vi "MenuSelection(User).vi"(6 "User events":T8, 7 "Clipboard":refnum<vi>, 8 "error in":errorcluster {"code" min=0 max=0}, 10 "ItemTag":string, 11 "Data in":T1={"Class"={"Ants"=refnum, "Layer"=refnum, "Templates"=refnum, "Icon"=refnum, "Glyph"=refnum, "Settings"=refnum, "Tools"=refnum, "History"=refnum}, "Ref"={"Add Layer"=refnum, "Remove Layer"=refnum, "Line Text"=[], "Body Text Spec"=refnum, "DNL_Font"=refnum, "glyph path str"=refnum, "templates path str"=refnum, "Arrow Up"=refnum, "Arrow Down"=refnum, "IE VI Ref"=refnum, "Glyphs tree"=refnum, "Templates tree"=refnum, "Layer Icon Text"=refnum, "Layer Template"=refnum, "Body Text"=refnum, "Search Templates"=refnum, "TextMarker"=refnum, "Tab Control"=refnum, "Search Glyphs"=refnum, "Line Color"=refnum, "DNL_Glyphs []"=refnum, "Fill Color"=refnum, "Tools"=refnum, "Icon"=refnum, "Preview"=refnum, "Ants"=refnum, "Terminals"=refnum, "menu reference"=refnum, "LayerNames"=[], "GlyphLoadAnimation"=refnum, "TemplateLoadAnimation"=refnum, "refreshGlyphs"=refnum, "refreshTemplates"=refnum}, "Support"={"AntsRect"={"left"=0, "top"=0, "right"=0, "bottom"=0}, "Mouse Move Coords"={"Horizontal"=0, "Vertical"=0}, "Mouse Down Coords"={"Horizontal"=0, "Vertical"=0}, "Temp Coord"={"Horizontal"=0, "Vertical"=0}, "Action"=enum."Default", "Edge Color"=4914962, "Fill Color"=16860, "Mouse Down?"=FALSE, "Draft Mode?"=FALSE, "Temp Icon"=bytes[3102], "CTRL Pressed"=FALSE, "Move Selection?"=FALSE, "AntsRect Orig"={"left"=0, "top"=0, "right"=0, "bottom"=0}, "Text"="", "TM Set?"=FALSE, "Mouse inside icon?"=FALSE, "Tool (old value)"=0, "Pencil Move Color"=0, "Swap Colors?"=FALSE, "Shift pressed?"=FALSE}}) -> (0 "error out":errorcluster {"code" min=0 max=0}, 3 "Data out":T1={"Class"={"Ants"=refnum, "Layer"=refnum, "Templates"=refnum, "Icon"=refnum, "Glyph"=refnum, "Settings"=refnum, "Tools"=refnum, "History"=refnum}, "Ref"={"Add Layer"=refnum, "Remove Layer"=refnum, "Line Text"=[], "Body Text Spec"=refnum, "DNL_Font"=refnum, "glyph path str"=refnum, "templates path str"=refnum, "Arrow Up"=refnum, "Arrow Down"=refnum, "IE VI Ref"=refnum, "Glyphs tree"=refnum, "Templates tree"=refnum, "Layer Icon Text"=refnum, "Layer Template"=refnum, "Body Text"=refnum, "Search Templates"=refnum, "TextMarker"=refnum, "Tab Control"=refnum, "Search Glyphs"=refnum, "Line Color"=refnum, "DNL_Glyphs []"=refnum, "Fill Color"=refnum, "Tools"=refnum, "Icon"=refnum, "Preview"=refnum, "Ants"=refnum, "Terminals"=refnum, "menu reference"=refnum, "LayerNames"=[], "GlyphLoadAnimation"=refnum, "TemplateLoadAnimation"=refnum, "refreshGlyphs"=refnum, "refreshTemplates"=refnum}, "Support"={"AntsRect"={"left"=0, "top"=0, "right"=0, "bottom"=0}, "Mouse Move Coords"={"Horizontal"=0, "Vertical"=0}, "Mouse Down Coords"={"Horizontal"=0, "Vertical"=0}, "Temp Coord"={"Horizontal"=0, "Vertical"=0}, "Action"=enum."Default", "Edge Color"=4914962, "Fill Color"=16860, "Mouse Down?"=FALSE, "Draft Mode?"=FALSE, "Temp Icon"=bytes[3102], "CTRL Pressed"=FALSE, "Move Selection?"=FALSE, "AntsRect Orig"={"left"=0, "top"=0, "right"=0, "bottom"=0}, "Text"="", "TM Set?"=FALSE, "Mouse inside icon?"=FALSE, "Tool (old value)"=0, "Pencil Move Color"=0, "Swap Colors?"=FALSE, "Shift pressed?"=FALSE}})   [LabVIEW 2020]
uses:
  Class/Ants/Ants.lvclass
  Class/FakedArray/FakedArray.lvclass
  vi.lib/LabVIEW Icon API/lv_icon/Classes/Icon/Icon.lvclass
  Class/Icon Library/Glyph.lvclass
  Class/Settings/Settings.lvclass
  Class/Tools/Tools Paint.lvclass
  History/History/History.lvclass
  vi.lib/LabVIEW Icon API/lv_icon/Classes/Icon Framework/Icon Framework.lvclass
  vi.lib/LabVIEW Icon API/lv_icon/Classes/Layer/Layer.lvclass
  vi.lib/LabVIEW Icon API/lv_icon/Controls/Layer.ctl
  Controls/Tools.ctl
  lv_icon.lvlib
  vi.lib/LabVIEW Icon API/LabVIEW Icon API.lvlib
  vi.lib/LabVIEW Icon API/lv_icon/Controls/Pathes.ctl
  History/History.lvlib
  vi.lib/LabVIEW Icon API/lv_icon/Controls/Graphic.ctl
  <vilib>/Utility/miscctls.llb/LVSelectionTypeDef.ctl
  <vilib>/Utility/miscctls.llb/LVPoint32TypeDef.ctl
  Controls/SupportClass_Action.ctl
  vi.lib/LabVIEW Icon API/lv_icon/Controls/IEColor.ctl
  Controls/Support Cluster.ctl
  Controls/References Cluster.ctl
  Controls/IE Classes.ctl
  Controls/Global Data.ctl
panel:
  in  "Layer name":string="Clipboard"
  in  "glyph":string="Glyph name"
  in  "template":string="Template name"
  in  "Prompt":string="Save Glyph"
  in  "prompt":string="Save Icon Template"
  in  "LayerName":string="Merged Layers"
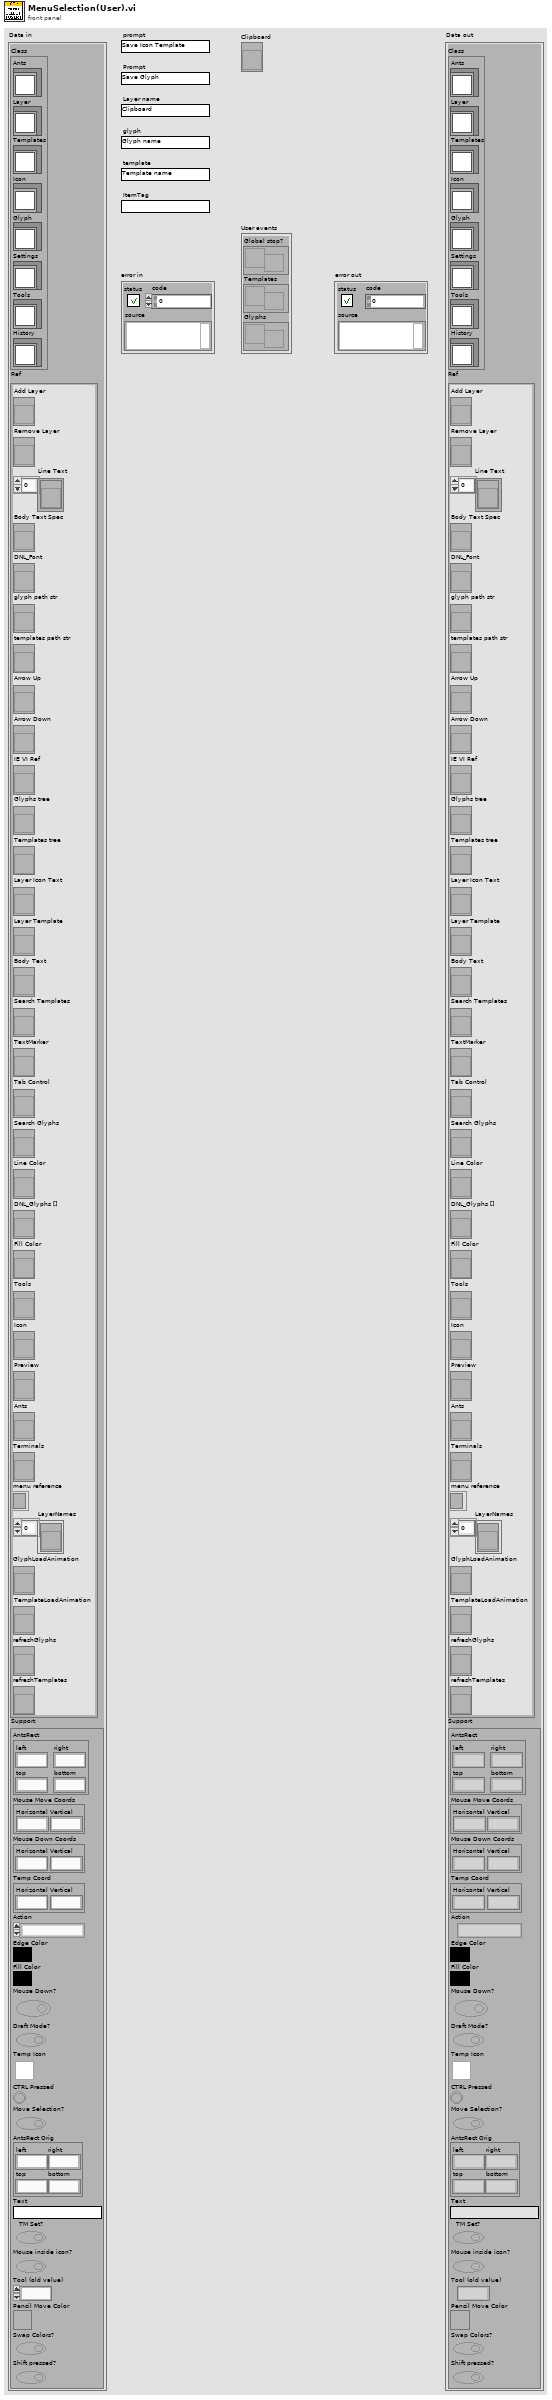
[diagram p1: front panel]
types:
  T1 = typedef "lv_icon.lvlib/Global Data.ctl" = cluster{"Class":T2, "Ref":T3, "Support":T4}
  T2 = typedef "lv_icon.lvlib/IE Classes.ctl" = cluster{"Ants":refnum<class "Ants.lvclass">, "Layer":refnum<class "FakedArray.lvclass">, "Templates":refnum<class "FakedArray.lvclass">, "Icon":refnum<class "Icon.lvclass">, "Glyph":refnum<class "Glyph.lvclass">, "Settings":refnum<class "Settings.lvclass">, "Tools":refnum<class "Tools Paint.lvclass">, "History":refnum<class "History.lvclass">}
  T3 = typedef "lv_icon.lvlib/References Cluster.ctl" = cluster{"Add Layer":refnum<vi>, "Remove Layer":refnum<vi>, "Line Text":refnum<vi>[], "Body Text Spec":refnum<vi>, "DNL_Font":refnum<vi>, "glyph path str":refnum<vi>, "templates path str":refnum<vi>, "Arrow Up":refnum<vi>, "Arrow Down":refnum<vi>, "IE VI Ref":refnum<vi>, "Glyphs tree":refnum<vi>, "Templates tree":refnum<vi>, "Layer Icon Text":refnum<vi>, "Layer Template":refnum<vi>, "Body Text":refnum<vi>, "Search Templates":refnum<vi>, "TextMarker":refnum<vi>, "Tab Control":refnum<vi>, "Search Glyphs":refnum<vi>, "Line Color":refnum<vi>, "DNL_Glyphs []":refnum<vi>, "Fill Color":refnum<vi>, "Tools":refnum<vi>, "Icon":refnum<vi>, "Preview":refnum<vi>, "Ants":refnum<vi>, "Terminals":refnum<vi>, "menu reference":refnum<k9>, "LayerNames":refnum<vi>[], "GlyphLoadAnimation":refnum<vi>, "TemplateLoadAnimation":refnum<vi>, "refreshGlyphs":refnum<vi>, "refreshTemplates":refnum<vi>}
  T4 = typedef "lv_icon.lvlib/Support Cluster.ctl" = cluster{"AntsRect":cluster{"left":i16, "top":i16, "right":i16, "bottom":i16}, "Mouse Move Coords":T5, "Mouse Down Coords":T5, "Temp Coord":T5, "Action":T6, "Edge Color":T7, "Fill Color":T7, "Mouse Down?":bool, "Draft Mode?":bool, "Temp Icon":picture, "CTRL Pressed":bool, "Move Selection?":bool, "AntsRect Orig":cluster{"left":i16, "top":i16, "right":i16, "bottom":i16}, "Text":string, "TM Set?":bool, "Mouse inside icon?":bool, "Tool (old value)":u32, "Pencil Move Color":u32, "Swap Colors?":bool, "Shift pressed?":bool}
  T5 = typedef "LVPoint32TypeDef.ctl" = cluster{"Horizontal":i32, "Vertical":i32}
  T6 = typedef "SupportClass_Action.ctl" = enum16{"Default", "Move Selection", "Glyph Library", "Tool"}
  T7 = typedef "IEColor.ctl" = u32
  T8 = cluster{"Global stop?":refnum<user-event>, "Templates":refnum<user-event>, "Glyphs":refnum<user-event>}
  T9 = typedef "Pathes.ctl" = enum16{"Root Path", "Icon Templates", "Icon Templates VI", "Icon Templates Lib", "Glyphs"}
  T10 = typedef "Graphic.ctl" = cluster{"Rectangle":cluster{"left":i16, "top":i16, "right":i16, "bottom":i16}, "Path":path, "Image":picture, "Filter":string, "FileName":string}
  T11 = typedef "Layer.ctl" = cluster{"LayerIcon":picture, "LayerName":string, "Opacity":u8, "Visibility?":bool}
  T12 = enum32{"Pencil", "Line", "Dropper", "Fill", "Rectangle", "Filled Rectangle", "Ellipse", "Filled Ellipse", "Eraser", "Text", "Select", "Move"}
  T13 = typedef "LVSelectionTypeDef.ctl" = cluster{"Selection Start":u32, "Selection End":u32}
  T14 = typedef "Tools.ctl" = enum32{"Pencil", "Line", "Dropper", "Fill", "Rectangle", "Filled Rectangle", "Ellipse", "Filled Ellipse", "Eraser", "Text", "Select", "Move"}
  T15 = typedef "imagedata.ctl" = cluster{"image type":i32, "image depth":i32, "image":u8[], "mask":u8[], "colors":u32[], "Rectangle":cluster{"left":i16, "top":i16, "right":i16, "bottom":i16}}
  T16 = typedef "Font.ctl" = string
  T17 = typedef "Alignment.ctl" = u16
  T18 = typedef "Font Size.ctl" = u8
  T19 = cluster{"Line 1 text":string, "Line 2 text":string, "Line 3 text":string, "Line 4 text":string, "Line 1 color":u32, "Line 2 color":u32, "Line 3 color":u32, "Line 4 color":u32, "Body Text Spec":cluster{"DNL_Font":T16, "Alignment":T17, "Size":T18}, "Center text vertically":bool, "Capitalize Text":bool}
  T20 = cluster{"left":i16, "top":i16, "right":i16, "bottom":i16}
  T21 = cluster{"Horizontal":i32, "Vertical":i32, "Vertical 2":i32, "Vertical 3":i32}
  T22 = typedef "lv_icon.lvlib/History.lvlib/State.ctl" = cluster{"Template":string, "Layers":string, "Body Text":string, "Icon Text Layer":string, "Template Layer":string, "Templates Search":string, "Glyphs Search":string}
  T23 = cluster{"Left":i32, "Top":i32, "Right":i32, "Bottom":i32}
  T24 = typedef "Icon Editor Invoker Type.ctl" = enum32{"Unknown Icon Source", "VI Icon", "Library Icon (any library type)", "Palette icon", "Icon from App Method"}
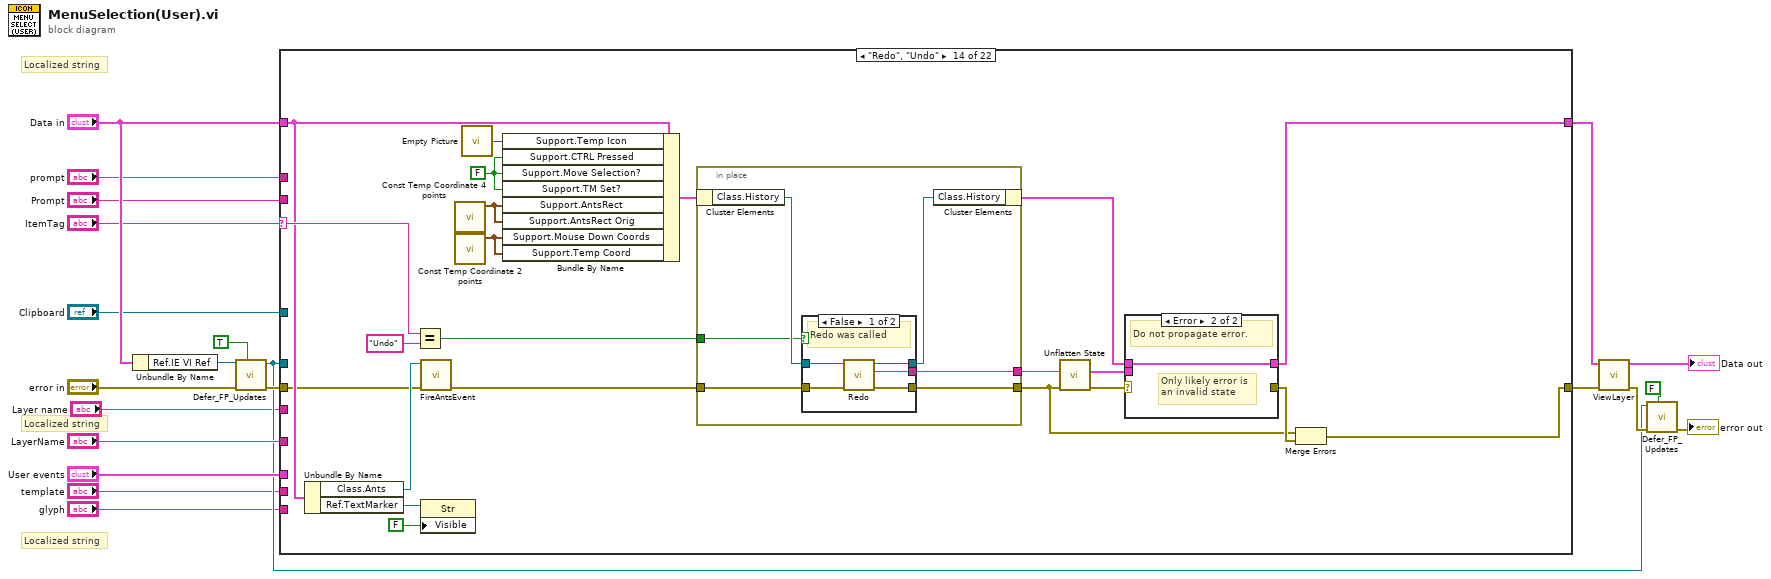
[diagram p0: block diagram]
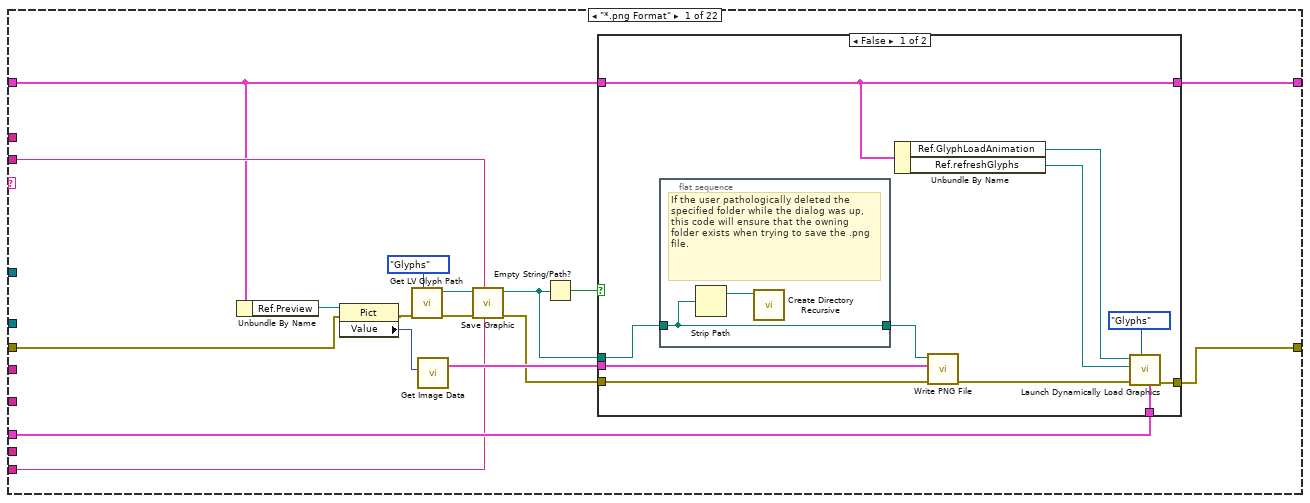
[diagram p2: hidden frame]
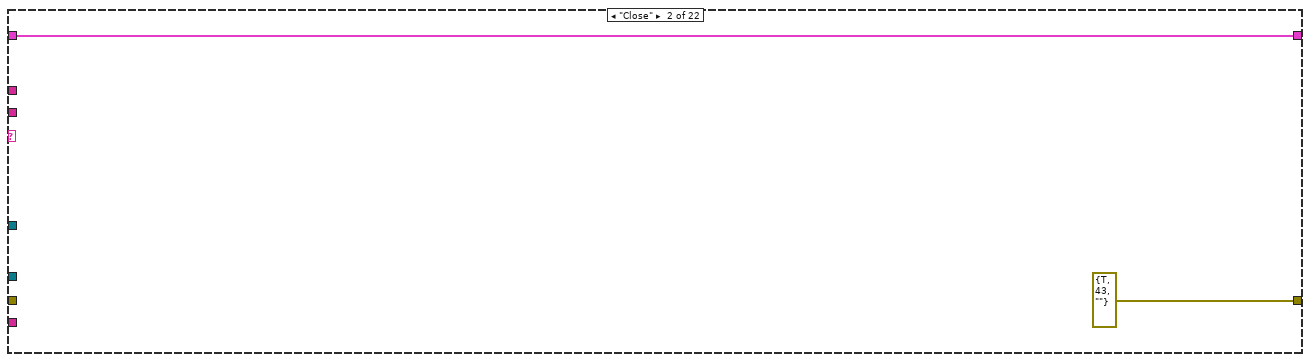
[diagram p4: hidden frame]
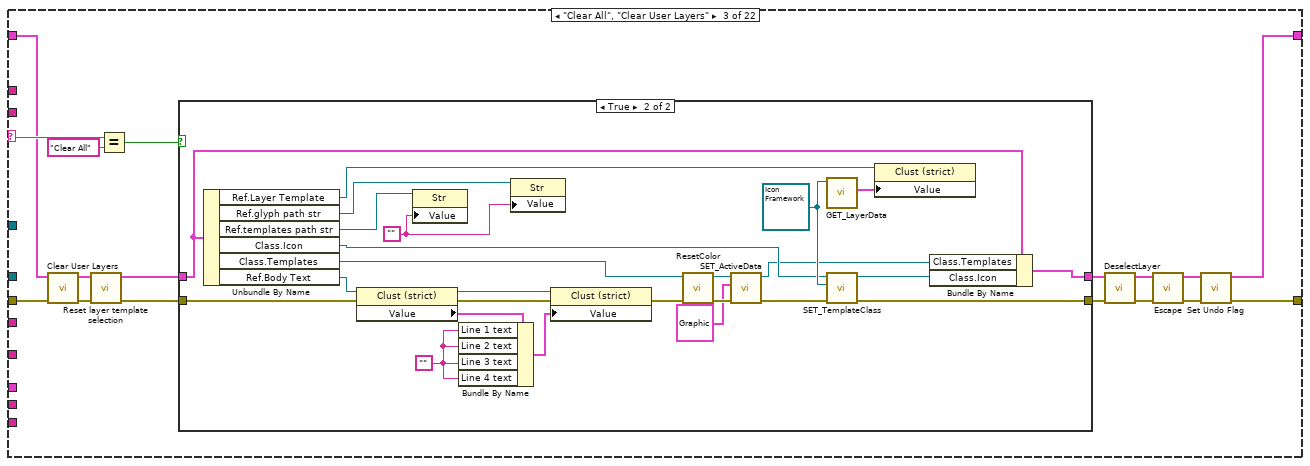
[diagram p5: hidden frame]
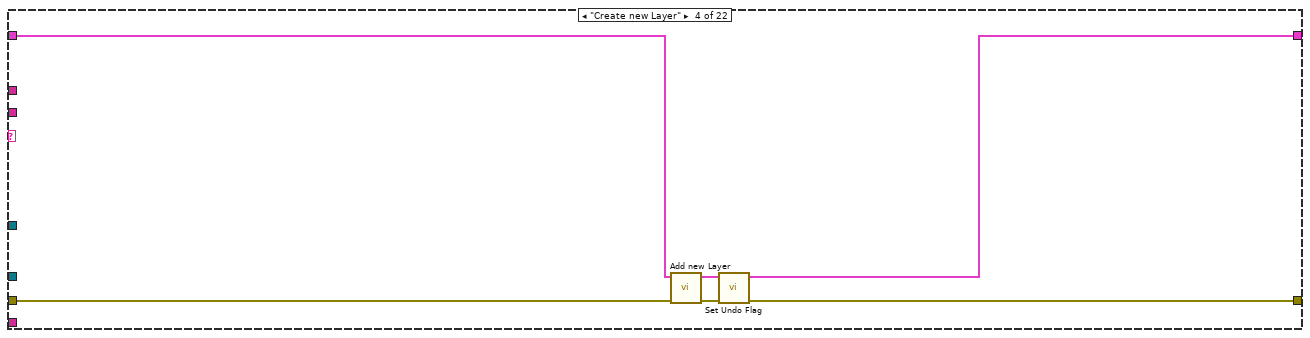
[diagram p7: hidden frame]
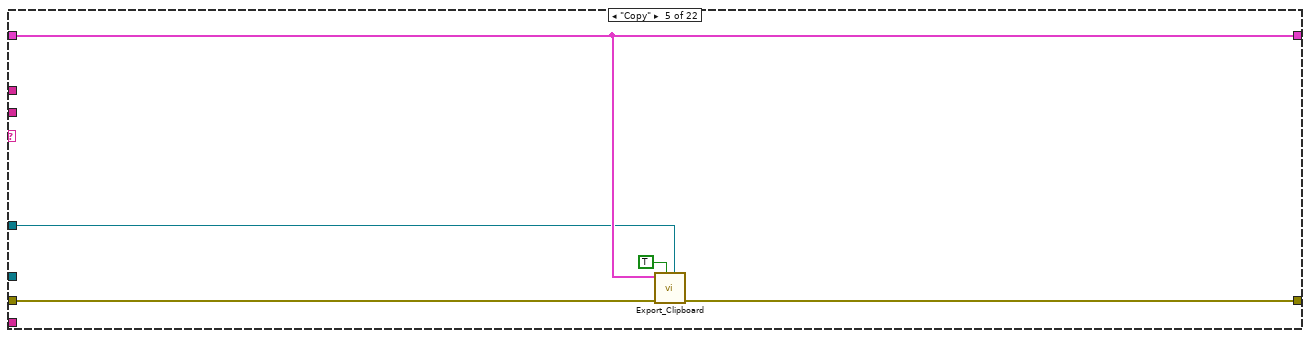
[diagram p8: hidden frame]
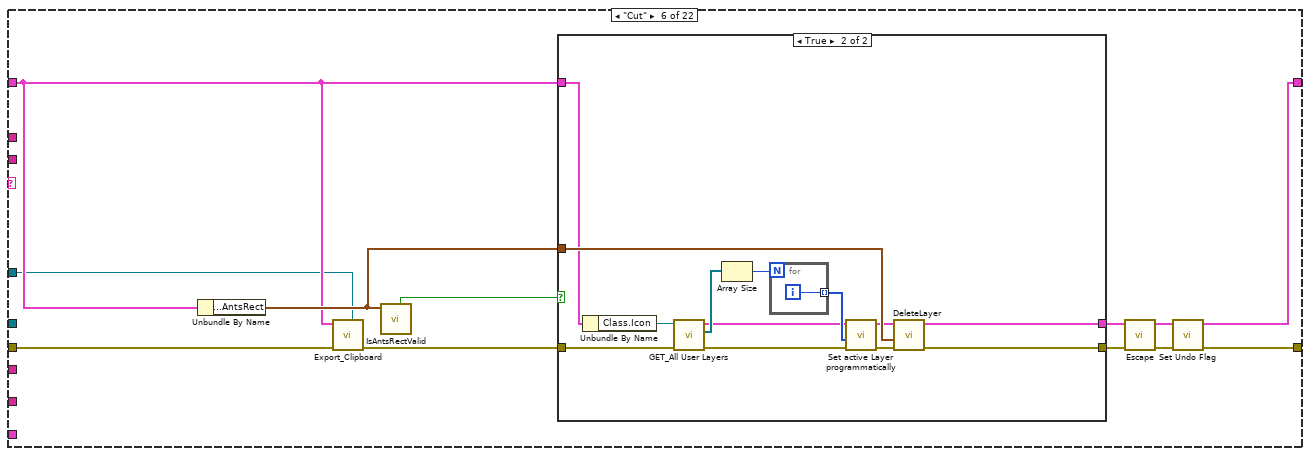
[diagram p9: hidden frame]
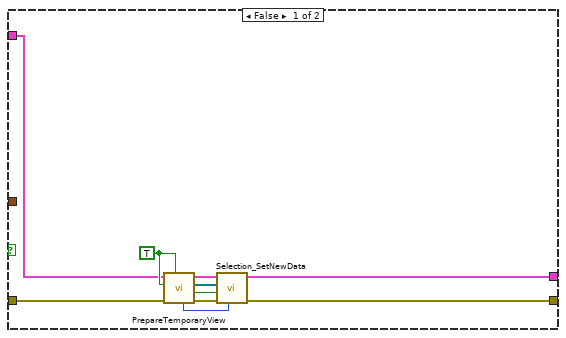
[diagram p10: hidden frame]
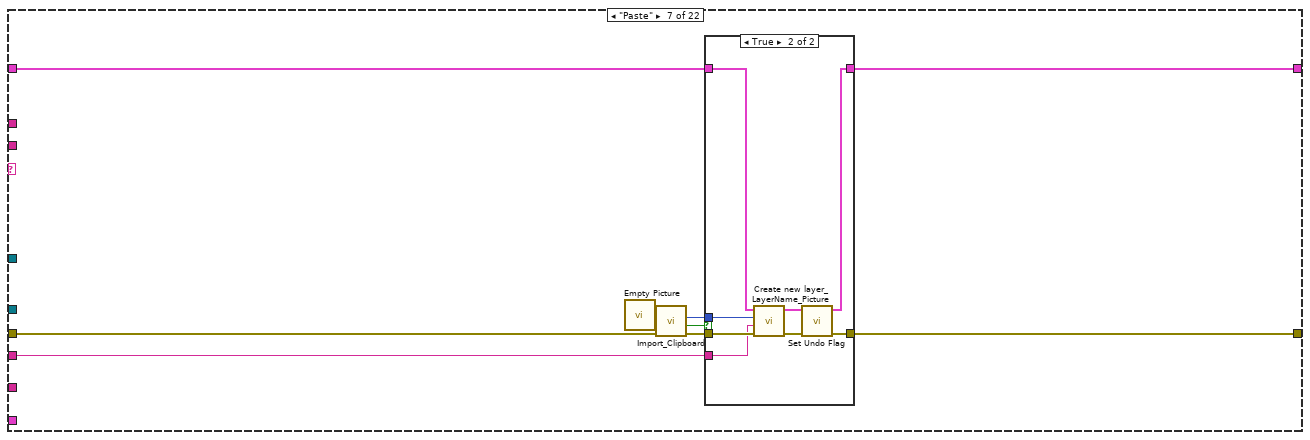
[diagram p11: hidden frame]
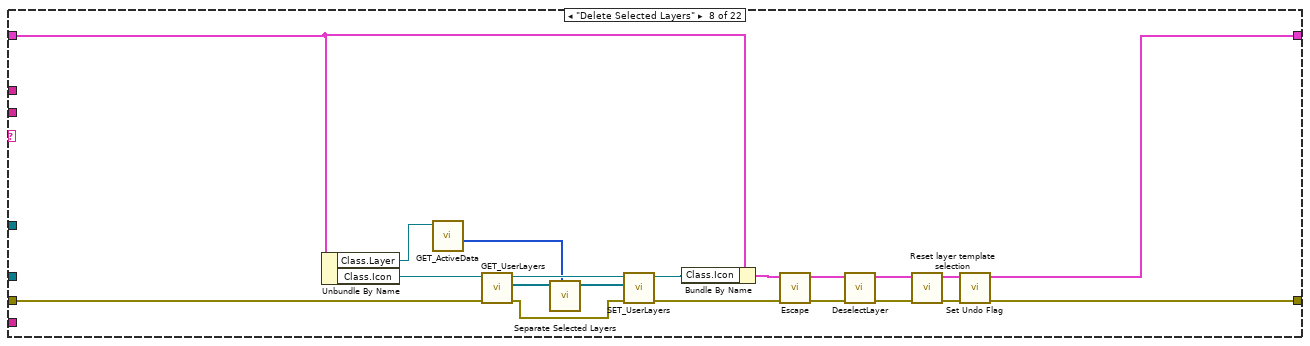
[diagram p13: hidden frame]
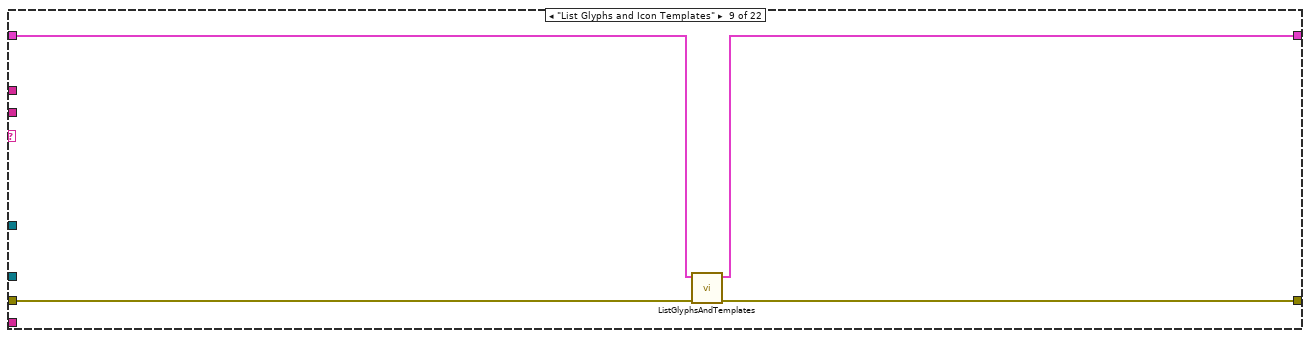
[diagram p14: hidden frame]
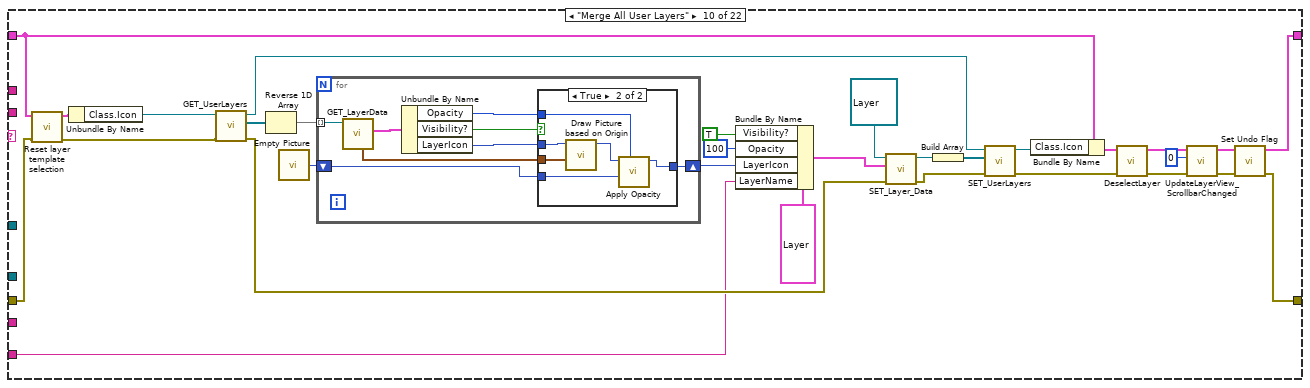
[diagram p15: hidden frame]
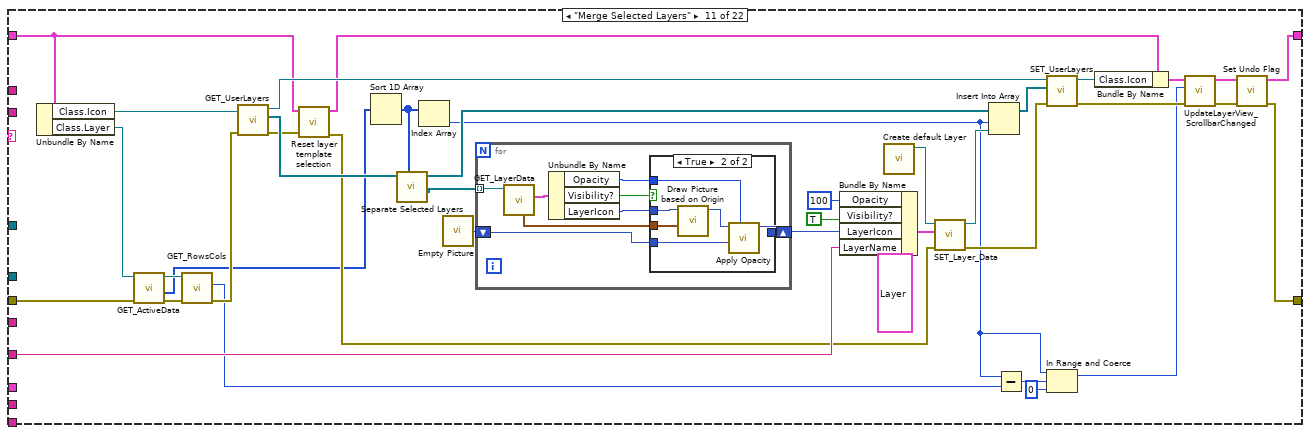
[diagram p17: hidden frame]
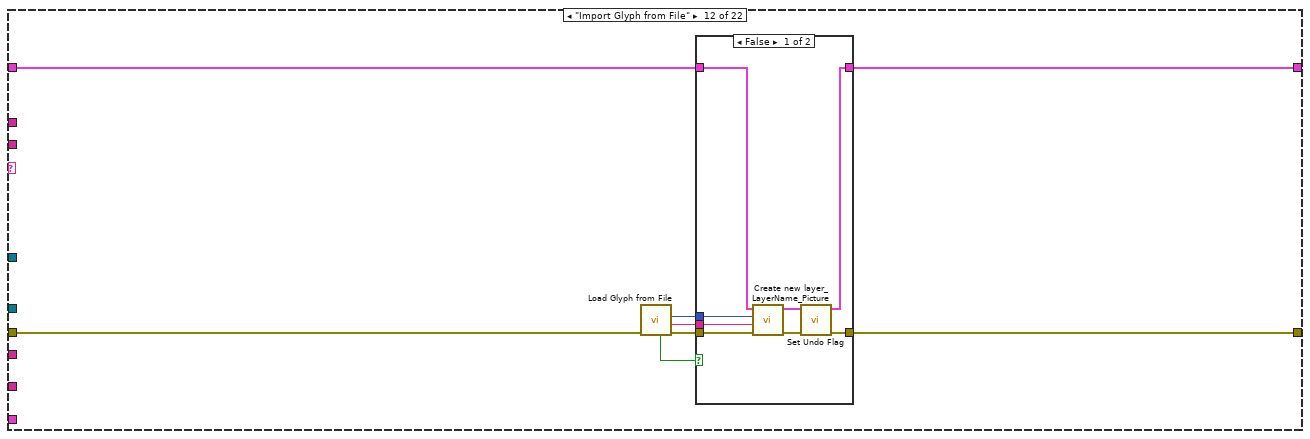
[diagram p19: hidden frame]
diagram:
  # "Localized string"
  # "Localized string"
  # "Localized string"
  n1 = Unbundle By Name("Data in") -> ("Ref.IE VI Ref"=w9:refnum<vi>)
  n2 = call "Defer_FP_Updates.vi"("Defer Panel Updates"=TRUE, "error in"="error in", "lv_icon.vi in"=w9) -> ("error out"=w11:errorcluster, "lv icon.vi out"=w5:refnum<vi>)  [unwired: 7 out]
  n3 = case shown="\"Redo\", \"Undo\"" "ItemTag" {
    selector: "ItemTag" -> [_ _ w72 _ _ _ _ _ _ _ _ _ _ w334 _ w415 _ _ _ _ _ _]
    tunnel: w11 -> [w26 _ w63 w103 w110 w117 w150 w177 w188 w205 w238 w292 w319 w330 w374 w406 w423 w425 w447 w469 w499 w504]
    tunnel: [w27 errorcluster {"status"=TRUE, "code"=43, "source"=""} ("Icon 43") w58 w102 w109 w113 w153 w167 w187 w191 w236 w294 w306 w324 w372 w408 w417 w426 w453 w468 w500 w504] -> w15
    tunnel: "LayerName" -> [_ _ _ _ _ _ _ _ _ w206 w261 _ _ _ _ _ _ _ _ _ _ _]
    tunnel: "prompt" -> [_ _ _ _ _ _ _ _ _ _ _ _ _ _ _ _ _ _ _ w471 _ _]
    tunnel: "Prompt" -> [w28 _ _ _ _ _ _ _ _ _ _ _ _ _ _ _ _ _ _ _ _ _]
    tunnel: "User events" -> [w33 _ _ _ _ _ _ _ _ _ _ _ _ _ _ _ _ _ w452 w477 _ _]
    tunnel: [w22 w54 w56 w100 w107 w111 w152 w165 w185 w189 w234 w293 w308 w329 w373 w407 w416 w424 w438 w464 w498 w503] -> w13
    tunnel: "Data in" -> [w23 w54 w64 w105 w107 w115 w154 w172 w186 w201 w254 w295 w311 w332 w369 w409 w422 w429 w439 w474 w498 w503]
    tunnel: w5 -> [_ _ _ _ _ _ _ _ _ _ _ _ _ _ _ _ _ _ _ _ w502 _]
    tunnel: "template" -> [_ _ _ _ _ _ _ _ _ _ _ _ _ _ _ _ _ _ _ w466 _ _]
    tunnel: "glyph" -> [w24 _ _ _ _ _ _ _ _ _ _ _ _ _ _ _ _ _ _ _ _ _]
    tunnel: "Layer name" -> [_ _ _ _ _ _ w146 _ _ _ _ _ _ _ _ _ _ _ _ _ _ _]
    tunnel: "Clipboard" -> [_ _ _ _ w106 w114 _ _ _ _ _ _ _ _ _ _ _ _ _ _ _ _]
    frame "*.png Format" {
      n4 = Unbundle By Name(w23) -> ("Ref.Preview"=w38:refnum<vi>)
      n5 = property class="Pict"(reference=w38, error in=w26) -> (error out=w34:errorcluster, "Value"=w36:picture)  [unwired: 1 out]
      n6 = call "Get LV Glyph Path.vi"("Path"=Pathes."Glyphs", "error in (no error)"=w34) -> ("error out"=w32:errorcluster, "Requested Path"=w29:path)  [unwired: 1 in, 7 out]
      n7 = call "Get Image Data.vi"("Pic In"=w36) -> ("image data out"=w37:T15)  [unwired: 3 in, 7 out]
      n8 = call "Save Graphic.vi"("Loc string caption"=w24, "FP Title"=w28, "error in (no error)"=w32, "Start path in"=w29) -> ("error out"=w31:errorcluster, "Output"=w30:path)  [unwired: 6 out]
      n9 = Empty String/Path?(string/path=w30) -> (empty?=w25:bool)
      n10 = case shown="False" w25 {
        tunnel: w37 -> [w49 _]
        tunnel: w33 -> [w46 _]
        tunnel: w31 -> [w45 w53]
        tunnel: w30 -> [w40 _]
        tunnel: [w44 w53] -> w27
        tunnel: w23 -> [w43 w52]
        tunnel: [w43 w52] -> w22
        frame False {
          n11 = flat-sequence {
            tunnel: w40 -> [w51]
            tunnel: [w51] -> w39
            frame #0 {
              # "If the user pathologically deleted the specified folder while the dialog was up, this code will ensure that the owning folder exists when trying to save the .png file."
              n12 = Strip Path(path=w51) -> (stripped path=w50:path)  [unwired: 1 out]
              n13 = call <vilib>:"Create Directory Recursive.vi"("directory"=w50) -> ()  [unwired: 4 in, 3 out]
            }
          }
          n14 = Unbundle By Name(w43) -> ("Ref.GlyphLoadAnimation"=w41:refnum<vi>, "Ref.refreshGlyphs"=w42:refnum<vi>)
          n15 = call <vilib>:"Write PNG File.vi"("error in (no error)"=w45, "image data"=w49, "path to PNG file"=w39) -> ("error out"=w48:errorcluster)  [unwired: 1 in, 7 out]
          n16 = call "Launch Dynamically Load Graphics.vi"("User events"=w46, "Path"=Pathes."Glyphs", "error in (no error)"=w48, "button ref"=w42, "animatedDecoration ref"=w41) -> ("error out"=w44:errorcluster)  [unwired: 1 in, 5 out]
        }
        frame True {
        }
      }
    }
    frame "Close" {
    }
    frame "Clear All", "Clear User Layers" {
      n17 = call "Clear User Layers.vi"("error in"=w63, "Data in"=w64) -> ("error out"=w62:errorcluster, "Data out"=w61:T1)  [unwired: 8 out]
      n18 = call "Reset layer template selection.vi"("error in (no error)"=w62, "Data in"=w61) -> ("error out"=w59:errorcluster, "Data out"=w60:T1)  [unwired: 1 in, 7 out]
      n19 = Equal?(x=w72, y="Clear All") -> (x = y?=w71:bool)
      n20 = case shown="True" w71 {
        tunnel: w59 -> [w74 w89]
        tunnel: w60 -> [w73 w81]
        tunnel: [w74 w84] -> w69
        tunnel: [w73 w82] -> w68
        frame False {
        }
        frame True {
          w99 = refnum<class "Icon Framework.lvclass"> refnum ("lv_icon.lvlib:Icon Framework.lvclass")
          w78 = ""
          w94 = ""
          n21 = Unbundle By Name(w81) -> ("Ref.Layer Template"=w76:refnum<vi>, "Ref.glyph path str"=w79:refnum<vi>, "Ref.templates path str"=w80:refnum<vi>, "Class.Icon"=w87:refnum<class "Icon.lvclass">, "Class.Templates"=w88:refnum<class "FakedArray.lvclass">, "Ref.Body Text"=w98:refnum<vi>)
          n22 = property class="Clust (strict)"(reference=w98, error in=w89) -> (reference out=w97:refnum<vi>, error out=w96:errorcluster, "Value"=w95:T19)
          n23 = property class="Str"(reference=w80, "Value"=w78) -> ()  [unwired: 1 in, 2 out]
          n24 = Bundle By Name(cluster=w95, "Line 1 text"=w94, "Line 2 text"=w94, "Line 3 text"=w94, "Line 4 text"=w94) -> (w90:T19)
          n25 = property class="Str"(reference=w79, "Value"=w78) -> ()  [unwired: 1 in, 2 out]
          n26 = property class="Clust (strict)"(reference=w97, error in=w96, "Value"=w90) -> (error out=w77:errorcluster)  [unwired: 1 out]
          n27 = call "ResetColor.vi"("error in (no error)"=w77, "FakedArray in"=w88) -> ("error out"=w92:errorcluster, "FakedArray out"=w93:refnum<class "FakedArray.lvclass">)  [unwired: 8 out]
          n28 = call-dynamic "SET_ActiveData.vi"("error in (no error)"=w92, "Active Data"=T10 {"Rectangle"={"left"=0, "top"=0, "right"=0, "bottom"=0}, "Path"=path "", "Image"=bytes[0], "Filter"="", "FileName"=""} ("Path & Icon"), "FakedArray.lvclass in"=w93) -> ("error out"=w86:errorcluster, "FakedArray.lvclass out"=w83:refnum<class "FakedArray.lvclass">)  [unwired: 7 out]
          n29 = call-dynamic "GET_LayerData.vi"("Layer.lvclass in"=w99) -> ("Data"=w75:T11)  [unwired: 1 in, 9 out]
          n30 = call-dynamic "SET_TemplateClass.vi"("error in (no error)"=w86, "Icon Framework.lvclass"=w99, "Icon.lvclass in"=w87) -> ("error out"=w84:errorcluster, "Icon.lvclass out"=w85:refnum<class "Icon.lvclass">)  [unwired: 7 out]
          n31 = property class="Clust (strict)"(reference=w76, "Value"=w75) -> ()  [unwired: 1 in, 2 out]
          n32 = Bundle By Name(cluster=w81, "Class.Templates"=w83, "Class.Icon"=w85) -> (w82:T1)
        }
      }
      n33 = call "DeselectLayer.vi"("error in (no error)"=w69, "Data in"=w68) -> ("error out"=w65:errorcluster, "Data out"=w67:T1)  [unwired: 8 out]
      n34 = call "Escape.vi"("error in"=w65, "Data in"=w67) -> ("error out"=w66:errorcluster, "Data out"=w57:T1)  [unwired: 2 in, 6 out]
      n35 = call "Set Undo Flag.vi"("error in"=w66, "Data in"=w57) -> ("error out"=w58:errorcluster, "Data out"=w56:T1)  [unwired: 8 in]
    }
    frame "Create new Layer" {
      n36 = call "Add new Layer.vi"("error in"=w103, "Data in"=w105) -> ("error out"=w104:errorcluster, "Data out"=w101:T1)  [unwired: 8 out]
      n37 = call "Set Undo Flag.vi"("error in"=w104, "Data in"=w101) -> ("error out"=w102:errorcluster, "Data out"=w100:T1)  [unwired: 8 in]
    }
    frame "Copy" {
      n38 = call "Export_Clipboard.vi"("Clipboard"=w106, "Is Copy? (F)"=TRUE, "error in"=w110, "Data in"=w107) -> ("error out"=w109:errorcluster)  [unwired: 1 in, 6 out]
    }
    frame "Cut" {
      n39 = Unbundle By Name(w115) -> ("Support.AntsRect"=w119:T20)
      n40 = call "Export_Clipboard.vi"("Clipboard"=w114, "error in"=w117, "Data in"=w115) -> ("error out"=w120:errorcluster)  [unwired: 1 in, 7 out]
      n41 = call "IsAntsRectValid.vi"("AntsRect"=w119) -> ("Max. Rect size?"=w121:bool)  [unwired: 10 out]
      n42 = case shown="True" w121 {
        tunnel: [w132 w143] -> w116
        tunnel: [w131 w144] -> w118
        tunnel: w120 -> [w124 w135]
        tunnel: w119 -> [_ w142]
        tunnel: w115 -> [w123 w133]
        frame False {
          w130 = TRUE ("Delete Selected Area?")
          n43 = call "PrepareTemporaryView.vi"("Delete Selected Area?"=w130, "error in (no error)"=w124, "Valid Selection?"=w130, "Data in"=w123) -> ("error out"=w127:errorcluster, "Highlighted?"=w128:bool, "All Layers out"=w129:refnum<class "Layer.lvclass">[], "Data out"=w125:T1, "#Active Layer"=w126:i32)  [unwired: 1 in, 2 out]
          n44 = call "Selection_SetNewData.vi"("#Active Layer"=w126, "error in"=w127, "Highlighted?"=w128, "All Layers In"=w129, "Data in"=w125) -> ("error out"=w132:errorcluster, "Data out"=w131:T1)  [unwired: 1 in, 3 out]
        }
        frame True {
          n45 = Unbundle By Name(w133) -> ("Class.Icon"=w141:refnum<class "Icon.lvclass">)
          n46 = call-dynamic "GET_All User Layers.vi"("error in (no error)"=w135, "Icon.lvclass in"=w141) -> ("error out"=w140:errorcluster, "User Layer"=w137:refnum<class "Layer.lvclass">[])  [unwired: 7 in, 1 out]
          n47 = Array Size(array=w137) -> (size(s)=w138:i32)
          n48 = for {
            N: w138 -> [_]
            tunnel: [w145] -> w139 mode=indexing
            i -> [w145]
          }
          n49 = call "Set active Layer programmatically.vi"("error in"=w140, "Active Layer []"=w139, "Data in"=w133) -> ("error out"=w134:errorcluster, "Data out"=w136:T1)  [unwired: 7 in]
          n50 = call "DeleteLayer.vi"("error in"=w134, "AntsRect"=w142, "Data in"=w136) -> ("error out"=w143:errorcluster, "Data out"=w144:T1)  [unwired: 5 out]
        }
      }
      n51 = call "Escape.vi"("error in"=w116, "Data in"=w118) -> ("error out"=w122:errorcluster, "Data out"=w112:T1)  [unwired: 2 in, 6 out]
      n52 = call "Set Undo Flag.vi"("error in"=w122, "Data in"=w112) -> ("error out"=w113:errorcluster, "Data out"=w111:T1)  [unwired: 8 in]
    }
    frame "Paste" {
      n53 = call "Empty Picture"() -> ("empty picture"=w151:picture)
      n54 = call "Import_Clipboard.vi"("error in (no error)"=w150, "Picture in"=w151) -> ("error out"=w149:errorcluster, "Valid?"=w148:bool, "Picture"=w147:picture)  [unwired: 1 in, 6 out]
      n55 = case shown="True" w148 {
        tunnel: w154 -> [w155 w164]
        tunnel: [w156 w159] -> w153
        tunnel: [w155 w157] -> w152
        tunnel: w149 -> [w156 w162]
        tunnel: w147 -> [_ w161]
        tunnel: w146 -> [_ w160]
        frame False {
        }
        frame True {
          n56 = call "Create new layer_LayerName_Picture.vi"("error in"=w162, "Layer name"=w160, "Picture"=w161, "Data in"=w164) -> ("error out"=w163:errorcluster, "Data out"=w158:T1)  [unwired: 6 in]
          n57 = call "Set Undo Flag.vi"("error in"=w163, "Data in"=w158) -> ("error out"=w159:errorcluster, "Data out"=w157:T1)  [unwired: 8 in]
        }
      }
    }
    frame "Delete Selected Layers" {
      n58 = Unbundle By Name(w172) -> ("Class.Layer"=w170:refnum<class "FakedArray.lvclass">, "Class.Icon"=w180:refnum<class "Icon.lvclass">)
      n59 = call-dynamic "GET_ActiveData.vi"("FakedArray in"=w170) -> ("Active Data []"=w178:i32[])  [unwired: 1 in, 9 out]
      n60 = call-dynamic "GET_UserLayers.vi"("error in (no error)"=w177, "Icon.lvclass in"=w180) -> ("error out"=w181:errorcluster, "All Layers"=w184:refnum<class "Layer.lvclass">[], "Icon.lvclass out"=w183:refnum<class "Icon.lvclass">)  [unwired: 7 out]
      n61 = call "Separate Selected Layers.vi"("Active Indices"=w178, "All Layers"=w184) -> ("Layers out not in Array"=w182:refnum<class "Layer.lvclass">[])  [unwired: 9 out]
      n62 = call-dynamic "SET_UserLayers.vi"("error in"=w181, "Layers"=w182, "Icon.lvclass in"=w183) -> ("error out"=w169:errorcluster, "Icon.lvclass out"=w179:refnum<class "Icon.lvclass">)  [unwired: 7 in]
      n63 = Bundle By Name(cluster=w172, "Class.Icon"=w179) -> (w171:T1)
      n64 = call "Escape.vi"("error in"=w169, "Data in"=w171) -> ("error out"=w176:errorcluster, "Data out"=w175:T1)  [unwired: 8 out]
      n65 = call "DeselectLayer.vi"("error in (no error)"=w176, "Data in"=w175) -> ("error out"=w173:errorcluster, "Data out"=w174:T1)  [unwired: 8 out]
      n66 = call "Reset layer template selection.vi"("error in (no error)"=w173, "Data in"=w174) -> ("error out"=w168:errorcluster, "Data out"=w166:T1)  [unwired: 1 in, 7 out]
      n67 = call "Set Undo Flag.vi"("error in"=w168, "Data in"=w166) -> ("error out"=w167:errorcluster, "Data out"=w165:T1)  [unwired: 8 in]
    }
    frame "List Glyphs and Icon Templates" {
      n68 = call "ListGlyphsAndTemplates.vi"("error in"=w188, "Data in"=w186) -> ("error out"=w187:errorcluster, "Data out"=w185:T1)  [unwired: 8 out]
    }
    frame "Merge All User Layers" {
      n69 = call "Reset layer template selection.vi"("error in (no error)"=w205, "Data in"=w201) -> ("error out"=w204:errorcluster, "Data out"=w203:T1)  [unwired: 1 in, 7 out]
      n70 = Unbundle By Name(w203) -> ("Class.Icon"=w202:refnum<class "Icon.lvclass">)
      n71 = call-dynamic "GET_UserLayers.vi"("error in (no error)"=w204, "Icon.lvclass in"=w202) -> ("error out"=w210:errorcluster, "All Layers"=w218:refnum<class "Layer.lvclass">[], "Icon.lvclass out"=w217:refnum<class "Icon.lvclass">)  [unwired: 7 out]
      n72 = Reverse 1D Array(array=w218) -> (reversed array=w208:refnum<class "Layer.lvclass">[])
      n73 = call "Empty Picture"() -> ("empty picture"=w207:picture)
      n74 = for {
        shift-right: [w223] -> w214
        shift-left: w207 -> [w224]
        tunnel: w208 -> [w219] mode=indexing
        n75 = call-dynamic "GET_LayerData.vi"("Layer.lvclass in"=w219) -> ("Data"=w221:T11, "Origin"=w220:T5)  [unwired: 1 in, 8 out]
        n76 = Unbundle By Name(w221) -> ("Opacity"=w225:u8, "Visibility?"=w226:bool, "LayerIcon"=w222:picture)
        n77 = case shown="True" w226 {
          tunnel: w225 -> [_ w233]
          tunnel: w224 -> [w227 w232]
          tunnel: [w227 w231] -> w223
          tunnel: w222 -> [_ w230]
          tunnel: w220 -> [_ w229]
          frame False {
          }
          frame True {
            n78 = call "Draw Picture based on Origin.vi"("Origin"=w229, "LayerIcon in"=w230) -> ("LayerIcon out"=w228:picture)  [unwired: 1 in, 8 out]
            n79 = call "Apply Opacity.vi"("% (100)"=w233, "Bottom"=w232, "Top"=w228) -> ("new picture"=w231:picture)  [unwired: 8 out]
          }
        }
      }
      n80 = Bundle By Name(cluster=T11 {"LayerIcon"=bytes[0], "LayerName"="", "Opacity"=0, "Visibility?"=FALSE} ("Data"), "Visibility?"=TRUE, "Opacity"=u8 100, "LayerIcon"=w214, "LayerName"=w206) -> (w213:T11)
      n81 = call-dynamic "SET_Layer_Data.vi"("error in (no error)"=w210, "Data"=w213, "Layer.lvclass in"=refnum<class "Layer.lvclass"> refnum) -> ("error out"=w211:errorcluster, "Layer.lvclass out"=w216:refnum<class "Layer.lvclass">)  [unwired: 1 in, 6 out]
      n82 = Build Array(w216) -> (w209:refnum<class "Layer.lvclass">[])
      n83 = call-dynamic "SET_UserLayers.vi"("error in"=w211, "Layers"=w209, "Icon.lvclass in"=w217) -> ("error out"=w199:errorcluster, "Icon.lvclass out"=w200:refnum<class "Icon.lvclass">)  [unwired: 7 in]
      n84 = Bundle By Name(cluster=w201, "Class.Icon"=w200) -> (w198:T1)
      n85 = call "DeselectLayer.vi"("error in (no error)"=w199, "Data in"=w198) -> ("error out"=w194:errorcluster, "Data out"=w195:T1)  [unwired: 8 out]
      n86 = call "UpdateLayerView_ScrollbarChanged.vi"("error in"=w194, "Scrollbar Position"=0, "Data in"=w195) -> ("error out"=w193:errorcluster, "Data out"=w190:T1)  [unwired: 7 out]
      n87 = call "Set Undo Flag.vi"("error in"=w193, "Data in"=w190) -> ("error out"=w191:errorcluster, "Data out"=w189:T1)  [unwired: 8 in]
    }
    frame "Merge Selected Layers" {
      n88 = Unbundle By Name(w254) -> ("Class.Icon"=w256:refnum<class "Icon.lvclass">, "Class.Layer"=w241:refnum<class "FakedArray.lvclass">)
      n89 = call-dynamic "GET_ActiveData.vi"("error in (no error)"=w238, "FakedArray in"=w241) -> ("error out"=w239:errorcluster, "Active Data []"=w237:i32[], "FakedArray out"=w240:refnum<class "FakedArray.lvclass">)  [unwired: 7 out]
      n90 = call-dynamic "GET_RowsCols.vi"("error in (no error)"=w239, "FakedArray.lvclass in"=w240) -> ("error out"=w249:errorcluster, "# Rows"=w248:i32)  [unwired: 8 out]
      n91 = call-dynamic "GET_UserLayers.vi"("error in (no error)"=w249, "Icon.lvclass in"=w256) -> ("error out"=w260:errorcluster, "All Layers"=w265:refnum<class "Layer.lvclass">[], "Icon.lvclass out"=w266:refnum<class "Icon.lvclass">)  [unwired: 7 out]
      n92 = call "Reset layer template selection.vi"("error in (no error)"=w260, "Data in"=w254) -> ("error out"=w259:errorcluster, "Data out"=w253:T1)  [unwired: 1 in, 7 out]
      n93 = Sort 1D Array(array=w237) -> (sorted array=w272:i32[])
      n94 = call "Separate Selected Layers.vi"("Active Indices"=w272, "All Layers"=w265) -> ("Layers out in Array"=w263:refnum<class "Layer.lvclass">[], "Layers out not in Array"=w264:refnum<class "Layer.lvclass">[])  [unwired: 8 out]
      n95 = Index Array(array=w272) -> (element=w246:i32)  [unwired: 1 in]
      n96 = call "Empty Picture"() -> ("empty picture"=w268:picture)
      n97 = for {
        shift-right: [w277] -> w270
        shift-left: w268 -> [w278]
        tunnel: w263 -> [w273] mode=indexing
        n98 = call-dynamic "GET_LayerData.vi"("Layer.lvclass in"=w273) -> ("Data"=w275:T11, "Origin"=w274:T5)  [unwired: 1 in, 8 out]
        n99 = Unbundle By Name(w275) -> ("Opacity"=w279:u8, "Visibility?"=w280:bool, "LayerIcon"=w276:picture)
        n100 = case shown="True" w280 {
          tunnel: w279 -> [_ w287]
          tunnel: w278 -> [w281 w286]
          tunnel: [w281 w285] -> w277
          tunnel: w276 -> [_ w284]
          tunnel: w274 -> [_ w283]
          frame False {
          }
          frame True {
            n101 = call "Draw Picture based on Origin.vi"("Origin"=w283, "LayerIcon in"=w284) -> ("LayerIcon out"=w282:picture)  [unwired: 1 in, 8 out]
            n102 = call "Apply Opacity.vi"("% (100)"=w287, "Bottom"=w286, "Top"=w282) -> ("new picture"=w285:picture)  [unwired: 8 out]
          }
        }
      }
      n103 = Bundle By Name(cluster=T11 {"LayerIcon"=bytes[0], "LayerName"="", "Opacity"=0, "Visibility?"=FALSE} ("Data"), "Opacity"=u8 100, "Visibility?"=TRUE, "LayerIcon"=w270, "LayerName"=w261) -> (w269:T11)
      n104 = call "Create default Layer.vi"() -> ("Layer.lvclass out"=w257:refnum<class "Layer.lvclass">)  [unwired: 1 in, 10 out]
      n105 = call-dynamic "SET_Layer_Data.vi"("error in (no error)"=w259, "Data"=w269, "Layer.lvclass in"=w257) -> ("error out"=w258:errorcluster, "Layer.lvclass out"=w267:refnum<class "Layer.lvclass">)  [unwired: 1 in, 6 out]
      n106 = Insert Into Array(array=w264, index=w246, new element=w267) -> (w262:refnum<class "Layer.lvclass">[])
      n107 = Subtract(x=w246, y=w248) -> (x-y=w247:i32)
      n108 = call-dynamic "SET_UserLayers.vi"("error in"=w258, "Layers"=w262, "Icon.lvclass in"=w266) -> ("error out"=w251:errorcluster, "Icon.lvclass out"=w255:refnum<class "Icon.lvclass">)  [unwired: 7 in]
      n109 = In Range and Coerce(upper limit=w246, x=w247, lower limit=0) -> (coerced(x)=w244:i32)  [unwired: 1 out]
      n110 = Bundle By Name(cluster=w253, "Class.Icon"=w255) -> (w252:T1)
      n111 = call "UpdateLayerView_ScrollbarChanged.vi"("error in"=w251, "Scrollbar Position"=w244, "Data in"=w252) -> ("error out"=w250:errorcluster, "Data out"=w235:T1)  [unwired: 7 out]
      n112 = call "Set Undo Flag.vi"("error in"=w250, "Data in"=w235) -> ("error out"=w236:errorcluster, "Data out"=w234:T1)  [unwired: 8 in]
    }
    frame "Import Glyph from File" {
      n113 = call "Load Glyph from File.vi"("error in (no error)"=w292) -> ("error out"=w291:errorcluster, "file name"=w288:string, "Pic Out"=w289:picture, "Canceled?"=w290:bool)  [unwired: 7 in]
      n114 = case shown="False" w290 {
        tunnel: w295 -> [w301 w304]
        tunnel: [w298 w305] -> w294
        tunnel: [w296 w304] -> w293
        tunnel: w291 -> [w303 w305]
        tunnel: w289 -> [w299 _]
        tunnel: w288 -> [w300 _]
        frame False {
          n115 = call "Create new layer_LayerName_Picture.vi"("error in"=w303, "Layer name"=w300, "Picture"=w299, "Data in"=w301) -> ("error out"=w302:errorcluster, "Data out"=w297:T1)  [unwired: 6 in]
          n116 = call "Set Undo Flag.vi"("error in"=w302, "Data in"=w297) -> ("error out"=w298:errorcluster, "Data out"=w296:T1)  [unwired: 8 in]
        }
        frame True {
        }
      }
    }
    frame "Import Icon from Owning Library" {
      n117 = Unbundle By Name(w311) -> ("Class.Icon"=w318:refnum<class "Icon.lvclass">)
      n118 = call "Read Data from Caller.vi"("error in (no error)"=w319) -> ("error out"=w317:errorcluster, "Library Icon"=w315:picture)  [unwired: 5 in, 4 out]
      n119 = call-dynamic "GET_UserLayers.vi"("error in (no error)"=w317, "Icon.lvclass in"=w318) -> ("error out"=w312:errorcluster, "All Layers"=w316:refnum<class "Layer.lvclass">[], "Icon.lvclass out"=w314:refnum<class "Icon.lvclass">)  [unwired: 7 out]
      n120 = call "Create or Substitute NI_Layer layer.vi"("All Layers in"=w316, "new picture"=w315) -> ("All Layers out"=w313:refnum<class "Layer.lvclass">[])
      n121 = call-dynamic "SET_UserLayers.vi"("error in"=w312, "Layers"=w313, "Icon.lvclass in"=w314) -> ("error out"=w307:errorcluster, "Icon.lvclass out"=w310:refnum<class "Icon.lvclass">)  [unwired: 7 in]
      n122 = Bundle By Name(cluster=w311, "Class.Icon"=w310) -> (w309:T1)
      n123 = call "Set Undo Flag.vi"("error in"=w307, "Data in"=w309) -> ("error out"=w306:errorcluster, "Data out"=w308:T1)  [unwired: 8 in]
    }
    frame "Redo", "Undo" {
      w338 = FALSE ("TM Set?")
      n124 = Unbundle By Name(w332) -> ("Class.Ants"=w331:refnum<class "Ants.lvclass">, "Ref.TextMarker"=w336:refnum<vi>)
      n125 = Equal?(x=w334, y="Undo") -> (x = y?=w327:bool)
      n126 = call "FireAntsEvent.vi"("error in (no error)"=w330, "Ants in"=w331) -> ("error out"=w328:errorcluster)  [unwired: 2 in, 7 out]
      n127 = property class="Str"(reference=w336, "Visible"=FALSE) -> ()  [unwired: 1 in, 2 out]
      n128 = call "Const Temp Coordinate 4 points.vi"() -> ("Const Temp Coordinate"=w340:T21)  [unwired: 11 out]
      n129 = call "Const Temp Coordinate 2 points.vi"() -> ("Const Temp Coordinate"=w339:T5)  [unwired: 11 out]
      n130 = call "Empty Picture"() -> ("empty picture"=w337:picture)
      n131 = Bundle By Name(cluster=w332, "Support.Temp Icon"=w337, "Support.CTRL Pressed"=w338, "Support.Move Selection?"=w338, "Support.TM Set?"=w338, "Support.AntsRect"=w340, "Support.AntsRect Orig"=w340, "Support.Mouse Down Coords"=w339, "Support.Temp Coord"=w339) -> (w326:T1)
      n132 = in-place {
        in-place-border: w328 -> [w347]
        in-place-border: w327 -> [w342]
        in-place-border: [w344] -> w323
        in-place-border: [w343] -> w321
        n133 = in-place-cluster #1(w326) -> ("Class.History"=w346:refnum<class "History.lvclass">)
        n134 = case shown="False" w342 {
          tunnel: w347 -> [w349 w357]
          tunnel: w346 -> [w352 w356]
          tunnel: [w351 w355] -> w345
          tunnel: [w350 w354] -> w344
          tunnel: [w348 w353] -> w343
          frame False {
            # "Redo was called"
            n135 = call "Redo.vi"("error in"=w349, "History in"=w352) -> ("error out"=w350:errorcluster, "State"=w348:string, "History out"=w351:refnum<class "History.lvclass">)  [unwired: 7 in]
          }
          frame True {
            # "Undo was called"
            n136 = call "Undo.vi"("error in"=w357, "History in"=w356) -> ("error out"=w354:errorcluster, "State"=w353:string, "History out"=w355:refnum<class "History.lvclass">)  [unwired: 7 in]
          }
        }
        n137 = in-place-cluster #1("Class.History"=w345) -> (w325:T1)
      }
      n138 = call "Unflatten State.vi"("error in"=w323, "Flattened State"=w321) -> ("error out"=w322:errorcluster, "State"=w320:T22)  [unwired: 8 in]
      n139 = case shown="Error" w322 {
        selector: w322 -> [w361 _]
        tunnel: [w362 _] -> w341
        tunnel: w325 -> [w360 w363]
        tunnel: [w359 w363] -> w329
        tunnel: w320 -> [w358 _]
        frame No Error {
          # "Set the state of editor."
          n140 = call "Set to State.vi"("error in"=w361, "State"=w358, "Data in"=w360) -> ("error out"=w362:errorcluster, "Data out"=w359:T1)  [unwired: 5 in, 2 out]
        }
        frame Error {
          # "Only likely error is\nan invalid state"
          # "Do not propagate error."
        }
      }
      n141 = Merge Errors(w323, w341) -> (w324:errorcluster)
    }
    frame "Select All" {
      n142 = Unbundle By Name(w369) -> ("Ref.Search Templates"=w368:refnum<vi>, "Ref.Line Text"=w367:refnum<vi>[], "Ref.Search Glyphs"=w366:refnum<vi>, "Ref.LayerNames"=w365:refnum<vi>[])
      n143 = Build Array (concatenate)(w368, w367, w366, w365) -> (w364:refnum<vi>[])
      n144 = for {
        tunnel: w364 -> [w405] mode=indexing
        tunnel: [w404] -> w370
        tunnel: [w403] -> w371
        stop <- w403 stop-if-true
        n145 = property class="Str"(reference=w405) -> (reference out=w404:refnum<vi>, "Key Focus"=w403:bool)  [unwired: 1 in, 1 out]
      }
      n146 = case shown="False" w371 {
        tunnel: w374 -> [w394 w398]
        tunnel: w369 -> [w379 w399]
        tunnel: [w381 w399] -> w373
        tunnel: [w380 w401] -> w372
        tunnel: w370 -> [_ w402]
        frame False {
          w396 = T23 {"Left"=0, "Top"=0, "Right"=32, "Bottom"=32} ("Rectangle")
          # "String control does not have focus"
          n147 = Unbundle By Name(w379) -> ("Class.Icon"=w378:refnum<class "Icon.lvclass">, "Class.Ants"=w377:refnum<class "Ants.lvclass">, "Ref.Tools"=w376:refnum<vi>, "Ref.Ants"=w375:refnum<vi>)
          n148 = property class="Pict"(reference=w375, error in=w394, "Visible"=TRUE) -> (error out=w389:errorcluster)  [unwired: 1 out]
          n149 = property class="RadioBtnsControl (strict)"(reference=w376, error in=w389, "Value"=T12."Select" ("Value (Signaling)")) -> (error out=w390:errorcluster)  [unwired: 1 out]
          n150 = call "Const Temp Coordinate 2 points.vi"() -> ("Const Temp Coordinate"=w393:T5)  [unwired: 11 out]
          n151 = Bundle By Name(cluster=w379, "Support.CTRL Pressed"=FALSE, "Support.Tool (old value)"=u32 111, "Support.Mouse Move Coords"=w393, "Support.Mouse Down Coords"=w393, "Support.AntsRect"=w396, "Support.AntsRect Orig"=w396) -> (w382:T1)
          n152 = call "FireAntsEvent.vi"("error in (no error)"=w390, "Rectangle (default: deselect)"=w396, "Ants in"=w377) -> ("error out"=w387:errorcluster)  [unwired: 1 in, 7 out]
          n153 = call-dynamic "GET_All User Layers.vi"("error in (no error)"=w387, "Icon.lvclass in"=w378) -> ("error out"=w383:errorcluster, "User Layer"=w386:refnum<class "Layer.lvclass">[])  [unwired: 7 in, 1 out]
          n154 = Array Size(array=w386) -> (size(s)=w385:i32)
          n155 = for {
            N: w385 -> [_]
            tunnel: [w397] -> w384 mode=indexing
            i -> [w397]
          }
          n156 = call "Set active Layer programmatically.vi"("error in"=w383, "Active Layer []"=w384, "Data in"=w382) -> ("error out"=w380:errorcluster, "Data out"=w381:T1)  [unwired: 7 in]
        }
        frame True {
          # "Text Control is being edited. Select all text inside that control."
          n157 = property class="Str"(reference=w402, error in=w398, "Text.Selection"=T13 {"Selection Start"=0, "Selection End"=4294967295}) -> (error out=w401:errorcluster)  [unwired: 1 out]
        }
      }
    }
    frame "Select Font", "Settings" {
      n158 = Equal?(x=w415, y="Select Font") -> (x = y?=w413:bool)
      n159 = Select(t="Text" ("y"), s=w413, f="") -> (s? t:f=w410:string)
      n160 = call "IconEditorSettings.vi"("error in (no error)"=w406, "Active Tag"=w410, "Data in"=w409) -> ("error out"=w408:errorcluster, "Data out"=w407:T1)  [unwired: 7 out]
    }
    frame "Select None" {
      n161 = call "Escape.vi"("error in"=w423, "Data in"=w422) -> ("error out"=w418:errorcluster, "Data out"=w419:T1)  [unwired: 2 in, 6 out]
      n162 = call "DeselectLayer.vi"("error in (no error)"=w418, "Data in"=w419) -> ("error out"=w421:errorcluster, "Data out"=w420:T1)  [unwired: 8 out]
      n163 = call "Reset layer template selection.vi"("error in (no error)"=w421, "Data in"=w420) -> ("error out"=w417:errorcluster, "Data out"=w416:T1)  [unwired: 1 in, 7 out]
    }
    frame "Show Terminals" {
      n164 = Unbundle By Name(w429) -> ("Class.Settings"=w430:refnum<class "Settings.lvclass">)
      n165 = call-dynamic "GET_Show.vi"("error in"=w425, "Settings.lvclass in"=w430) -> ("error out"=w435:errorcluster, "Show Terminals?"=w432:bool, "Settings.lvclass out"=w437:refnum<class "Settings.lvclass">)  [unwired: 7 out]
      n166 = Not(x=w432) -> (.not. x?=w433:bool)
      n167 = call "ShowTerminals.vi"("Set Pic? (T)"=TRUE, "error in"=w435, "Tag enabled?"=TRUE, "Show Terminals?"=w433, "Data in"=w429) -> ("error out"=w434:errorcluster, "Data out"=w428:T1)  [unwired: 1 in, 4 out]
      n168 = call-dynamic "SET_Show.vi"("error in"=w434, "Show Terminals?"=w433, "Settings.lvclass in"=w437) -> ("error out"=w426:errorcluster, "Settings.lvclass out"=w427:refnum<class "Settings.lvclass">)  [unwired: 1 in, 6 out]
      n169 = Bundle By Name(cluster=w428, "Class.Settings"=w427) -> (w424:T1)
    }
    frame "Synchronize with Icon Library" {
      n170 = vi-ref "ni.com_iconlibrary.vi"() -> (w449:refnum<vi>)
      n171 = property class="VI"(reference=w449, error in=w447) -> (error out=w446:errorcluster, "Path"=w448:path)  [unwired: 1 out]
      n172 = Open VI Reference(vi path=w448, error in (no error)=w446) -> (vi reference=w450:refnum<vi>, error out=w451:errorcluster)  [unwired: 4 in]
      n173 = invoke class="VI" method="Run VI"(reference=w450, error in=w451, "Wait until done"=TRUE ("Wait Until Done"), "Auto Dispose Ref"=FALSE ("Auto Dispose Reference")) -> (reference out=w442:refnum<vi>, error out=w443:errorcluster)  [unwired: 1 in, 3 out]
      n174 = Close Reference(reference=w442, error in (no error)=w443) -> (error out=w440:errorcluster)
      n175 = Unbundle By Name(w440) -> ("code"=w441:i32)
      n176 = case shown="0, Default" w441 {
        tunnel: [w459 errorcluster {"status"=FALSE, "code"=0, "source"=""} ("error out")] -> w453
        tunnel: w452 -> [w458 _]
        tunnel: w440 -> [w457 _]
        tunnel: w439 -> [w456 w461]
        tunnel: [w456 w461] -> w438
        frame 0, Default {
          n177 = Unbundle By Name(w456) -> ("Ref.GlyphLoadAnimation"=w454:refnum<vi>, "Ref.refreshGlyphs"=w455:refnum<vi>)
          n178 = call "Launch Dynamically Load Graphics.vi"("User events"=w458, "Path"=Pathes."Glyphs", "error in (no error)"=w457, "button ref"=w455, "animatedDecoration ref"=w454) -> ("error out"=w459:errorcluster)  [unwired: 1 in, 5 out]
        }
        frame 1039 {
          # "VI was aborted"
        }
      }
    }
    frame "Template" {
      n179 = call "DrawIcon.vi"("Tools"=Tools."Ellipse", "error in (no error)"=w469, "Data in"=w474) -> ("error out"=w480:errorcluster, "Icon"=w479:picture, "Data out"=w465:T1)  [unwired: 2 in, 4 out]
      n180 = call "Read Data from Caller.vi"() -> ("Icon Editor Invoker Type"=w476:T24)  [unwired: 3 in, 8 out]
      n181 = call "Specify Path Enum.vi"("Icon Editor Invoker Type"=w476) -> ("Path"=w475:T9)  [unwired: 10 out]
      n182 = call "Get LV Glyph Path.vi"("Path"=w475, "error in (no error)"=w480) -> ("error out"=w473:errorcluster, "Requested Path"=w470:path)  [unwired: 1 in, 7 out]
      n183 = call "Get Image Data.vi"("Pic In"=w479) -> ("image data out"=w478:T15)  [unwired: 3 in, 7 out]
      n184 = call "Save Graphic.vi"("Loc string caption"=w466, "FP Title"=w471, "error in (no error)"=w473, "Start path in"=w470) -> ("error out"=w472:errorcluster, "Output"=w463:path)  [unwired: 6 out]
      n185 = Empty String/Path?(string/path=w463) -> (empty?=w467:bool)
      n186 = case shown="False" w467 {
        tunnel: w478 -> [w493 _]
        tunnel: w477 -> [w490 _]
        tunnel: w475 -> [w484 _]
        tunnel: w472 -> [w489 w497]
        tunnel: w463 -> [w483 _]
        tunnel: [w488 w497] -> w468
        tunnel: w465 -> [w487 w496]
        tunnel: [w487 w496] -> w464
        frame False {
          n187 = flat-sequence {
            tunnel: w483 -> [w495]
            tunnel: [w495] -> w482
            frame #0 {
              # "If the user pathologically deleted the specified folder while the dialog was up, this code will ensure that the owning folder exists when trying to save the .png file."
              n188 = Strip Path(path=w495) -> (stripped path=w494:path)  [unwired: 1 out]
              n189 = call <vilib>:"Create Directory Recursive.vi"("directory"=w494) -> ()  [unwired: 4 in, 3 out]
            }
          }
          n190 = Unbundle By Name(w487) -> ("Ref.TemplateLoadAnimation"=w486:refnum<vi>, "Ref.refreshTemplates"=w485:refnum<vi>)
          n191 = call <vilib>:"Write PNG File.vi"("error in (no error)"=w489, "image data"=w493, "path to PNG file"=w482) -> ("error out"=w492:errorcluster)  [unwired: 1 in, 7 out]
          n192 = call "Launch Dynamically Load Graphics.vi"("User events"=w490, "Template saved?"=TRUE, "Path"=w484, "error in (no error)"=w492, "button ref"=w485, "animatedDecoration ref"=w486) -> ("error out"=w488:errorcluster)  [unwired: 5 out]
        }
        frame True {
        }
      }
    }
    frame "Show Block Diagram" {
      n193 = property class="VI"(reference=w502, error in=w499, "BDWin.Open"=TRUE ("Block Diagram Window:Open")) -> (error out=w500:errorcluster)  [unwired: 1 out]
    }
    frame Default {
    }
  }
  n194 = call "ViewLayer.vi"("error in (no error)"=w15, "Data in"=w13) -> ("error out"=w7:errorcluster, "Data out"=→"Data out":T1)  [unwired: 2 in, 6 out]
  n195 = call "Defer_FP_Updates.vi"("Defer Panel Updates"=FALSE, "error in"=w7, "lv_icon.vi in"=w5) -> ("error out"=→"error out":errorcluster)  [unwired: 8 out]
